vi "Write Call Duration.vi"(8 "error in (no error)":errorcluster, 10 "Call Duration [ms]":u32, 11 "Customer With Phone In":refnum<class "Customer With Phone.lvclass">) -> (0 "error out":errorcluster, 3 "Customer With Phone Out":refnum<class "Customer With Phone.lvclass">)   [LabVIEW 2020, in "Customer With Phone.lvclass"]
uses:
  Customer With Phone.lvclass
  Customer With Phone.lvclass/Customer With Phone.ctl
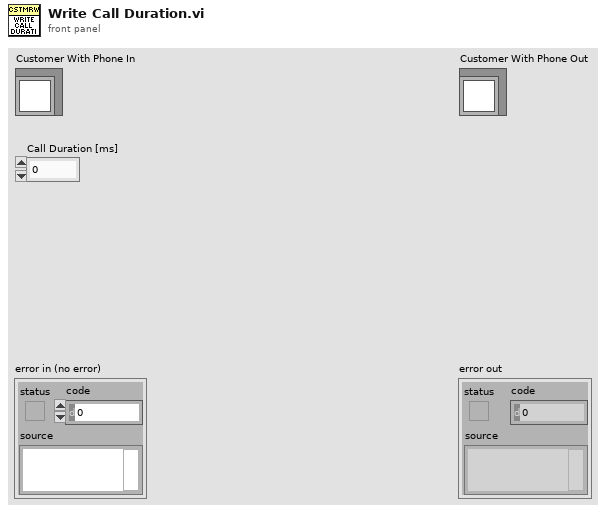
[diagram p1: front panel]
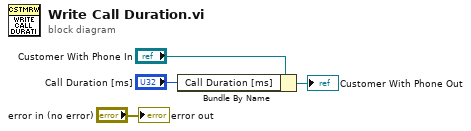
[diagram p0: block diagram]
diagram:
  n1 = Bundle By Name(cluster="Customer With Phone In", "Call Duration [ms]"="Call Duration [ms]") -> (→"Customer With Phone Out":refnum<class "Customer With Phone.lvclass">)
  "error out" <- "error in (no error)"
